vi "Forward Switch.vi"(8 "Command Info In":T1, 9 "Position":T5=enum."Far Right", 11 "Switch Position":T4) -> (0 "Command Info Out":T1)   [LabVIEW 2017]
uses:
  Support Code/Starting Position.ctl
  <vilib>/Rock Robotics/WPI/Framework/Completion Status.ctl
  <vilib>/Rock Robotics/WPI/Framework/Completion Notifier.ctl
  <vilib>/Rock Robotics/WPI/Framework/Command Status Info.ctl
  Support Code/Switch Position.ctl
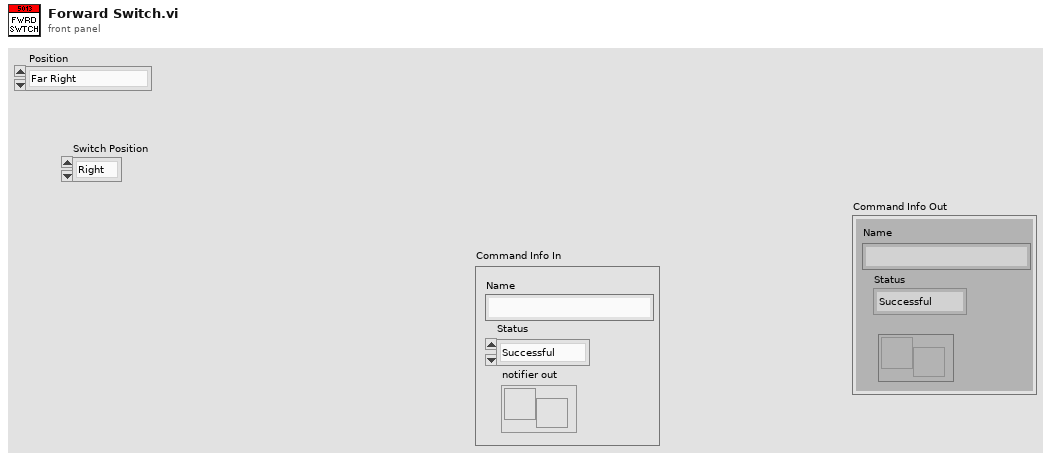
[diagram p1: front panel]
types:
  T1 = typedef "Command Status Info.ctl" = cluster{"Name":string, "Status":T2, "notifier out":T3}
  T2 = typedef "Completion Status.ctl" = enum16{"Successful", "Aborted", "Incomplete"}
  T3 = typedef "Completion Notifier.ctl" = refnum<notifier>
  T4 = typedef "Switch Position.ctl" = enum16{"Right", "Left"}
  T5 = typedef "Starting Position.ctl" = enum16{"Far Left", "Left", "Center", "Right", "Far Right"}
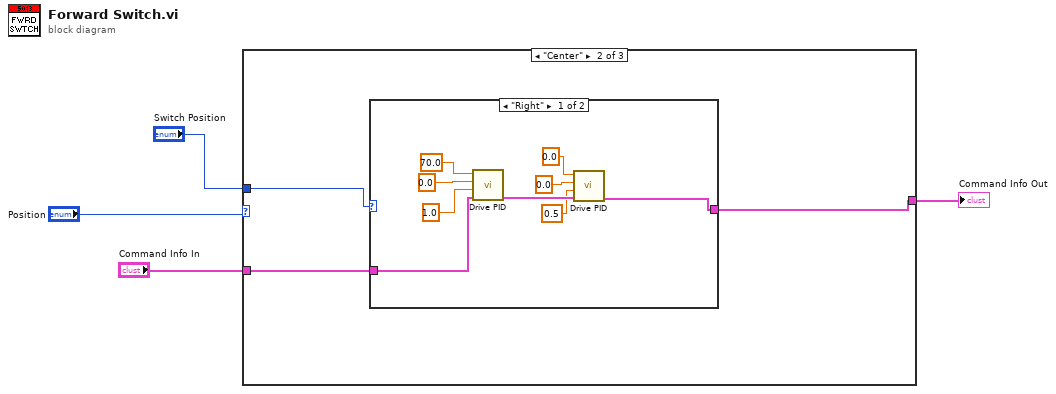
[diagram p0: block diagram]
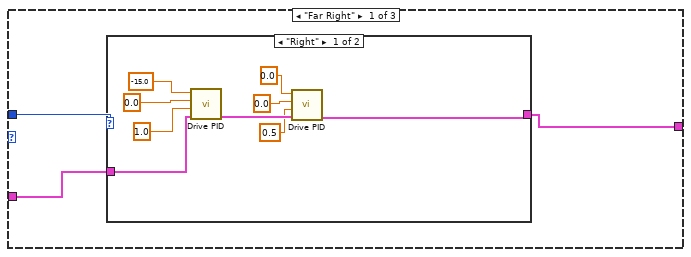
[diagram p2: hidden frame]
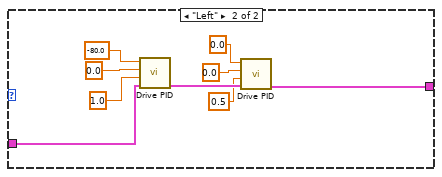
[diagram p3: hidden frame]
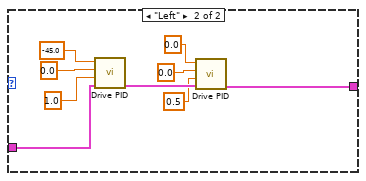
[diagram p4: hidden frame]
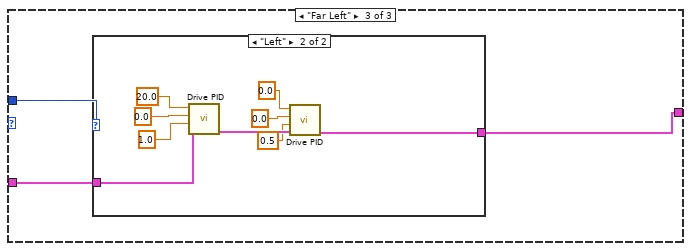
[diagram p5: hidden frame]
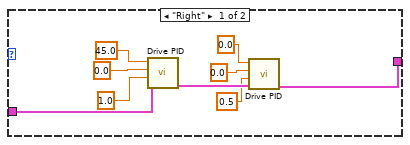
[diagram p6: hidden frame]
diagram:
  n1 = case shown="\"Center\"" "Position" {
    tunnel: "Command Info In" -> [w6 w28 w48]
    tunnel: "Switch Position" -> [w7 w27 w49]
    tunnel: [w5 w26 w47] -> w1
    frame "Far Right" {
      n2 = case shown="\"Right\"" w7 {
        tunnel: w6 -> [w9 w18]
        tunnel: [w8 w17] -> w5
        frame "Right" {
          n3 = call "Drive PID.vi"("Command Info In"=w9, "Speed"=1.0, "Distance"=0.0, "Target Angle"=-15.0) -> ("Command Info Out"=w14:T1)  [unwired: 7 in]
          n4 = call "Drive PID.vi"("Command Info In"=w14, "Speed"=0.5, "Distance"=0.0, "Target Angle"=0.0) -> ("Command Info Out"=w8:T1)  [unwired: 7 in]
        }
        frame "Left" {
          n5 = call "Drive PID.vi"("Command Info In"=w18, "Speed"=1.0, "Distance"=0.0, "Target Angle"=-80.0) -> ("Command Info Out"=w23:T1)  [unwired: 7 in]
          n6 = call "Drive PID.vi"("Command Info In"=w23, "Speed"=0.5, "Distance"=0.0, "Target Angle"=0.0) -> ("Command Info Out"=w17:T1)  [unwired: 7 in]
        }
      }
    }
    frame "Center" {
      n7 = case shown="\"Right\"" w27 {
        tunnel: w28 -> [w30 w39]
        tunnel: [w29 w38] -> w26
        frame "Right" {
          n8 = call "Drive PID.vi"("Command Info In"=w30, "Speed"=1.0, "Distance"=0.0, "Target Angle"=70.0) -> ("Command Info Out"=w35:T1)  [unwired: 7 in]
          n9 = call "Drive PID.vi"("Command Info In"=w35, "Speed"=0.5, "Distance"=0.0, "Target Angle"=0.0) -> ("Command Info Out"=w29:T1)  [unwired: 7 in]
        }
        frame "Left" {
          n10 = call "Drive PID.vi"("Command Info In"=w39, "Speed"=1.0, "Distance"=0.0, "Target Angle"=-45.0) -> ("Command Info Out"=w44:T1)  [unwired: 7 in]
          n11 = call "Drive PID.vi"("Command Info In"=w44, "Speed"=0.5, "Distance"=0.0, "Target Angle"=0.0) -> ("Command Info Out"=w38:T1)  [unwired: 7 in]
        }
      }
    }
    frame "Far Left" {
      n12 = case shown="\"Left\"" w49 {
        tunnel: w48 -> [w51 w60]
        tunnel: [w50 w59] -> w47
        frame "Right" {
          n13 = call "Drive PID.vi"("Command Info In"=w51, "Speed"=1.0, "Distance"=0.0, "Target Angle"=45.0) -> ("Command Info Out"=w56:T1)  [unwired: 7 in]
          n14 = call "Drive PID.vi"("Command Info In"=w56, "Speed"=0.5, "Distance"=0.0, "Target Angle"=0.0) -> ("Command Info Out"=w50:T1)  [unwired: 7 in]
        }
        frame "Left" {
          n15 = call "Drive PID.vi"("Command Info In"=w60, "Speed"=1.0, "Distance"=0.0, "Target Angle"=20.0) -> ("Command Info Out"=w65:T1)  [unwired: 7 in]
          n16 = call "Drive PID.vi"("Command Info In"=w65, "Speed"=0.5, "Distance"=0.0, "Target Angle"=0.0) -> ("Command Info Out"=w59:T1)  [unwired: 7 in]
        }
      }
    }
  }
  "Command Info Out" <- w1
